vi "get LED status.vi"(8 "error in (no error)":errorcluster, 11 "Cobolt in":refnum<class "Cobolt.lvclass">) -> (0 "error out":errorcluster, 1 "Laser":bool, 2 "Power":bool, 3 "Cobolt out":refnum<class "Cobolt.lvclass">, 4 "Error":bool, 5 "Lock":bool)   [LabVIEW 2012, in "Cobolt.lvclass"]
uses:
  Cobolt.lvclass
  CoboltLaserDrivers_Public_LV2012/CoboltLaser_Controls/ExpectedResponseType.ctl
  Cobolt.lvclass/Cobolt.ctl
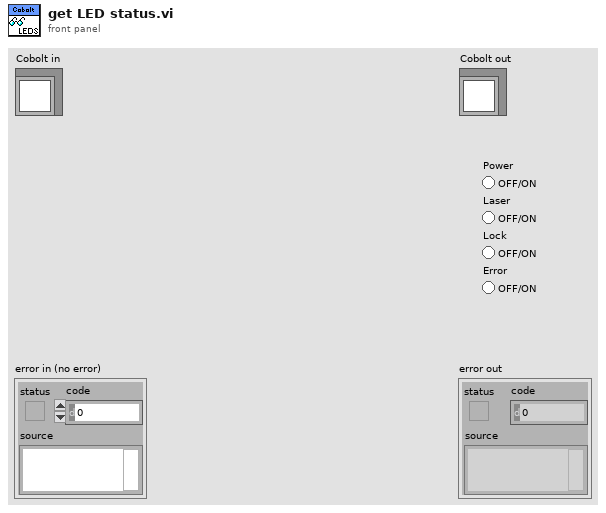
[diagram p1: front panel]
types:
  T1 = typedef "Cobolt.lvclass/ExpectedResponseType.ctl" = u16
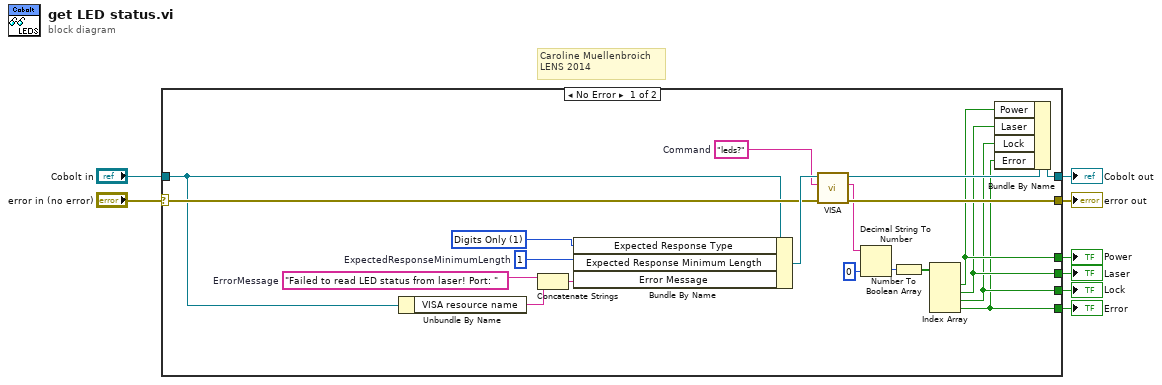
[diagram p0: block diagram]
diagram:
  # "Caroline Muellenbroich\nLENS 2014"
  n1 = case shown="No Error" "error in (no error)" {
    selector: "error in (no error)" -> [w20 w30]
    tunnel: [w21 w30] -> w7
    tunnel: [w19 w29] -> w5
    tunnel: "Cobolt in" -> [w18 w29]
    tunnel: [w12 _] -> w4
    tunnel: [w11 _] -> w3
    tunnel: [w9 _] -> w2
    tunnel: [w10 _] -> w1
    frame No Error {
      w22 = T1 1 items=["Any", "Digits Only", "Non-Digits Only"] ("ExpectedResponseType")
      w26 = 1  # ExpectedResponseMinimumLength
      w24 = "Failed to read LED status from laser! Port: "  # ErrorMessage
      w17 = "leds?"  # Command
      n2 = Unbundle By Name(w18) -> ("VISA resource name"=w25:string)
      n3 = Concatenate Strings(w24, w25) -> (w23:string)
      n4 = Bundle By Name(cluster=w18, "Expected Response Type"=w22, "Expected Response Minimum Length"=w26, "Error Message"=w23) -> (w27:refnum<class "Cobolt.lvclass">)
      n5 = call-dynamic "VISA.vi"("error in (no error)"=w20, "string to write"=w17, "Cobolt in"=w27) -> ("error out"=w21:errorcluster, "buffer out"=w13:string, "Cobolt out"=w28:refnum<class "Cobolt.lvclass">)  [unwired: 6 in]
      n6 = Decimal String To Number(string=w13, default (0L)=i16 0 ("default (0 I32)")) -> (number=w14:i16)  [unwired: 1 in, 1 out]
      n7 = Number To Boolean Array(number=w14) -> (Boolean array=w16:bool[])
      n8 = Index Array(array=w16) -> (element #1=w12:bool, element #2=w11:bool, element #3=w10:bool, element #4=w9:bool)  [unwired: 4 in]
      n9 = Bundle By Name(cluster=w28, "Power"=w12, "Laser"=w11, "Lock"=w10, "Error"=w9) -> (w19:refnum<class "Cobolt.lvclass">)
    }
    frame Error {
    }
  }
  "error out" <- w7
  "Cobolt out" <- w5
  "Power" <- w4
  "Laser" <- w3
  "Lock" <- w1
  "Error" <- w2
